vi "posi inicial-proceso 6.vi"() -> ()   [LabVIEW 2020]
panel:
  out "posi inicial-proceso 6":T1
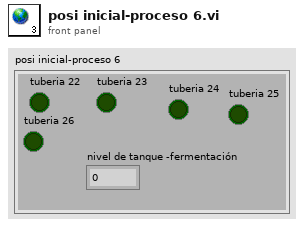
[diagram p1: front panel]
types:
  T1 = cluster{"tuberia 22":bool, "nivel de tanque -fermentación":dbl, "tuberia 23":bool, "tuberia 24":bool, "tuberia 25":bool, "tuberia 26":bool}
diagram:
